vi "Read Labels.vi"(8 "error in (no error)":errorcluster, 11 "Scanner in":refnum<class "Scanner.lvclass">) -> (0 "error out":errorcluster, 2 "Axis Label and Unit":T1, 3 "Scanner out":refnum<class "Scanner.lvclass">)   [LabVIEW 2009, in "Scanner.lvclass"]
uses:
  Scanner.lvclass
  Instruments/Utility Classes/Readable/Data Channel.ctl
  Instruments/Utility Classes/Readable/Data Point.ctl
  Scanner.lvclass/Scanner.ctl
  Instruments/Utility Classes/Scannable/Scannable.lvclass
  Instruments/Utility Classes/Readable/Readable.lvclass
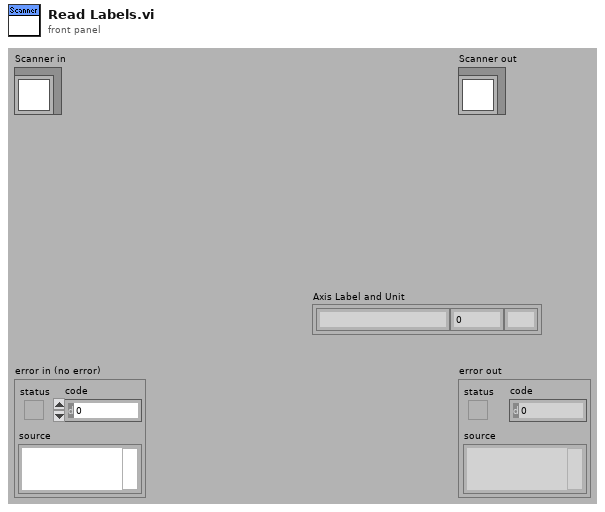
[diagram p1: front panel]
types:
  T1 = typedef "Readable.lvclass/Data Channel.ctl" = cluster{"Name":string, "Data Point":T2, "Unit":string}
  T2 = typedef "Readable.lvclass/Data Point.ctl" = dbl
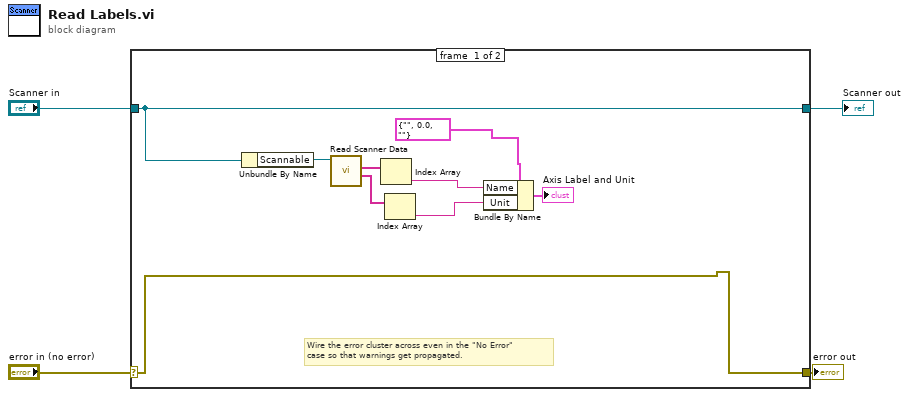
[diagram p0: block diagram]
diagram:
  n1 = case shown="No Error" "error in (no error)" {
    selector: "error in (no error)" -> [w13 w15]
    tunnel: [w13 w15] -> w3
    tunnel: [w11 w14] -> w1
    tunnel: "Scanner in" -> [w11 w14]
    frame #0 {
      # "Wire the error cluster across even in the \"No Error\"\ncase so that warnings get propagated."
      n2 = Unbundle By Name(w11) -> ("Scannable"=w12:refnum<class "Scannable.lvclass">)
      n3 = call-dynamic "Read Scanner Data.vi"("Scannable in"=w12) -> ("Channel Units"=w7:string[], "Channel Names"=w10:string[])  [unwired: 7 in, 2 out]
      n4 = Index Array(array=w10) -> (element=w9:string)  [unwired: 1 in]
      n5 = Index Array(array=w7) -> (element=w6:string)  [unwired: 1 in]
      n6 = Bundle By Name(cluster=T1 {"Name"="", "Data Point"=0.0, "Unit"=""} ("Add'l Data Channels"), "Name"=w9, "Unit"=w6) -> (→"Axis Label and Unit":T1)
    }
    frame #1 {
    }
  }
  "error out" <- w3
  "Scanner out" <- w1
